vi "cryo get numeric.vi"(5 "Bit array in":u8[](array[numeric])=[0, 0, 0, 0, 0, 0, 0, 0, 0, 0]) -> (4 "Numeric value out":dbl)   [LabVIEW 2009]
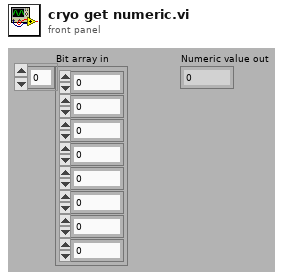
[diagram p1: front panel]
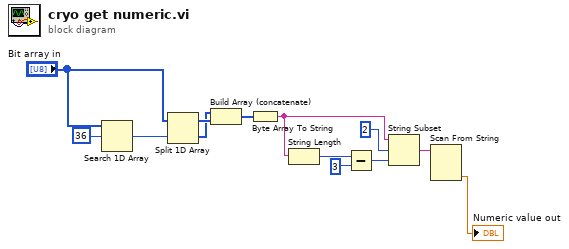
[diagram p0: block diagram]
diagram:
  n1 = Search 1D Array(1D array="Bit array in", element=u8 36) -> (index of element=w7:i32)  [unwired: 1 in]
  n2 = Split 1D Array(array="Bit array in", index=w7) -> (first subarray=w3:u8[], second subarray=w2:u8[])
  n3 = Build Array (concatenate)(w2, w3) -> (w4:u8[])
  n4 = Byte Array To String(unsigned byte array=w4) -> (string=w1:string)
  n5 = String Length(string=w1) -> (length=w9:i32)
  n6 = Subtract(x=w9, y=3) -> (x-y=w10:i32)
  n7 = String Subset(string=w1, offset (0)=2, length (rest)=w10) -> (substring=w12:string)
  n8 = Scan From String(input string=w12) -> (output 1=→"Numeric value out":dbl)  [unwired: 4 in, 3 out]
